vi "Read False.vi"(8 "Error In":errorcluster) -> (0 "Error Out":errorcluster)   [LabVIEW 2018, in "Tests.lvlib" / "Reader.lvlib"]
uses:
  Reader.lvlib
  src/Toolkit/Public/Reader/Private/Read False by Value.vi
  <vilib>/addons/_JKI Toolkits/Caraya/classes/Test/Test.lvclass
  <vilib>/addons/_JKI Toolkits/Caraya/classes/Assert/Assert.lvclass
  src/Toolkit/Public/Reader/Reader.lvclass
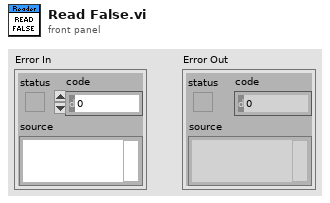
[diagram p1: front panel]
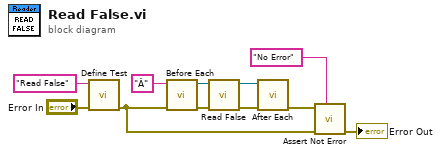
[diagram p0: block diagram]
diagram:
  n1 = call <vilib>:"Define Test.vi"("error in (no error)"="Error In", "Label (VI Title)"="Read False") -> ("error out"=w8:errorcluster)  [unwired: 9 in]
  n2 = call "Before Each.vi"("Error In"=w8, "Data"="Â") -> ("Error Out"=w3:errorcluster, "Reader"=w4:refnum<class "Reader.lvclass">)  [unwired: 8 in]
  n3 = call-poly "Read False.vi"("Error In"=w3, "Reader In"=w4) -> ("Error Out"=w6:errorcluster, "Reader Out"=w5:refnum<class "Reader.lvclass">)  [unwired: 8 in]
  n4 = call "After Each.vi"("Error In"=w6, "Reader In"=w5) -> ("Error Out"=w9:errorcluster)  [unwired: 9 in]
  n5 = call <vilib>:"Assert Not Error.vi"("Label"="No Error", "error in (no error)"=w8, "Not Error?"=w9) -> ("error out"=→"Error Out":errorcluster)  [unwired: 8 in]
